vi "Test Serialize Strings.vi"(8 "error in (no error)":errorcluster) -> (0 "error out":errorcluster)   [LabVIEW 2013]
uses:
  src/Serializer/JSON Serializer/JSON Serializer.lvclass
  <vilib>/addons/_JKI Toolkits/Caraya/classes/Test/Test.lvclass
  <vilib>/addons/_JKI Toolkits/Caraya/classes/Assert/Assert.lvclass
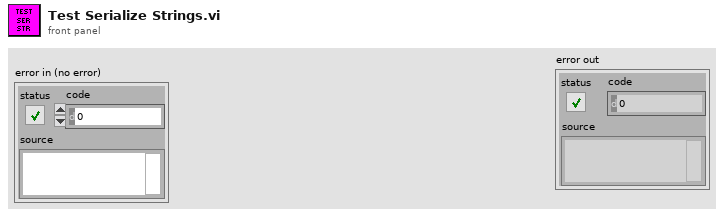
[diagram p1: front panel]
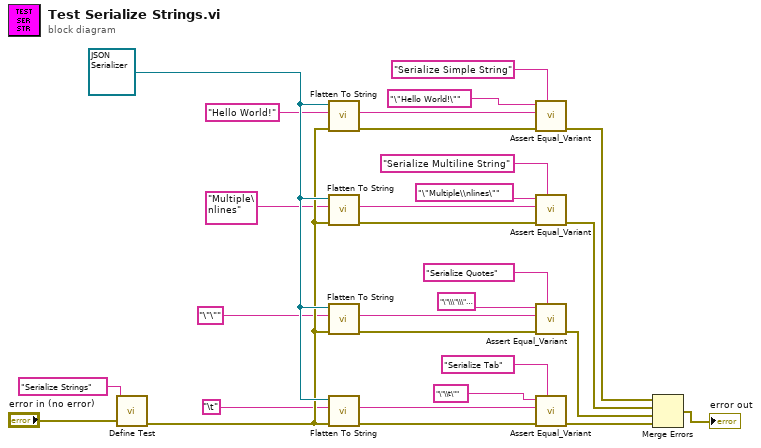
[diagram p0: block diagram]
diagram:
  w12 = refnum<class "JSON Serializer.lvclass"> refnum ("JKI JSON Serialization.lvlib:JSON Serializer.lvclass")
  n1 = call <vilib>:"Define Test.vi"("error in (no error)"="error in (no error)", "Label (VI Title)"="Serialize Strings") -> ("error out"=w11:errorcluster)  [unwired: 9 in]
  n2 = call-dynamic "Flatten To String.vi"("error in (no error)"=w11, "Variant"="Hello World!", "JSON Serializer in"=w12) -> ("error out"=w16:errorcluster, "String"=w15:string)  [unwired: 6 in, 1 out]
  n3 = call-dynamic "Flatten To String.vi"("error in (no error)"=w11, "Variant"="Multiple\nlines", "JSON Serializer in"=w12) -> ("error out"=w20:errorcluster, "String"=w19:string)  [unwired: 6 in, 1 out]
  n4 = call-dynamic "Flatten To String.vi"("error in (no error)"=w11, "Variant"="\"\"", "JSON Serializer in"=w12) -> ("error out"=w24:errorcluster, "String"=w23:string)  [unwired: 6 in, 1 out]
  n5 = call-dynamic "Flatten To String.vi"("error in (no error)"=w11, "Variant"="\t", "JSON Serializer in"=w12) -> ("error out"=w28:errorcluster, "String"=w27:string)  [unwired: 6 in, 1 out]
  n6 = call <vilib>:"Assert Equal_Variant.vi"("Label"="Serialize Simple String", "error in (no error)"=w16, "Y"=w15, "X"="\"Hello World!\"") -> ("error out"=w6:errorcluster)  [unwired: 7 in]
  n7 = call <vilib>:"Assert Equal_Variant.vi"("Label"="Serialize Multiline String", "error in (no error)"=w20, "Y"=w19, "X"="\"Multiple\\nlines\"") -> ("error out"=w7:errorcluster)  [unwired: 7 in]
  n8 = call <vilib>:"Assert Equal_Variant.vi"("Label"="Serialize Quotes", "error in (no error)"=w24, "Y"=w23, "X"="\"\\\"\\\"\"") -> ("error out"=w8:errorcluster)  [unwired: 7 in]
  n9 = call <vilib>:"Assert Equal_Variant.vi"("Label"="Serialize Tab", "error in (no error)"=w28, "Y"=w27, "X"="\"\\t\"") -> ("error out"=w9:errorcluster)  [unwired: 7 in]
  n10 = Merge Errors(w6, w7, w8, w9) -> (→"error out":errorcluster)
